vi "Simulated Database.vi"(11 "Command":T2) -> ()   [LabVIEW 2012]
uses:
  DataType/Simulated Database_Function.ctl
  DataType/Simulated Database_Record.ctl
panel:
  out "error out":errorcluster
  in  "error in (no error)":errorcluster
  out "owned record?":bool
  in  "Banlance or Account":i32
  out "Record":T1 {"Balance" format="%9.2f"; "Account Number" format="%0#5_5g"}
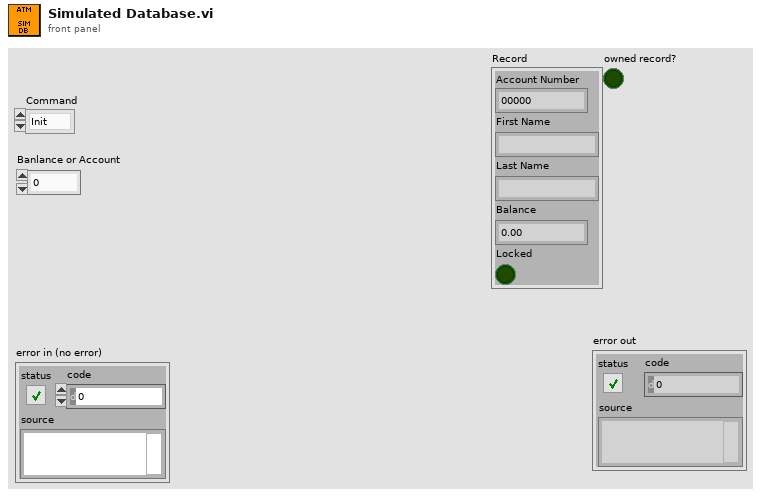
[diagram p1: front panel]
types:
  T1 = typedef "Simulated Database_Record.ctl" = cluster{"Account Number":dbl, "First Name":string, "Last Name":string, "Balance":dbl, "Locked":bool}
  T2 = typedef "Simulated Database_Function.ctl" = enum16{"Init", "Search account and lock record", "Modify balance", "Access record", "Commit record", "Unlock record", "Close"}
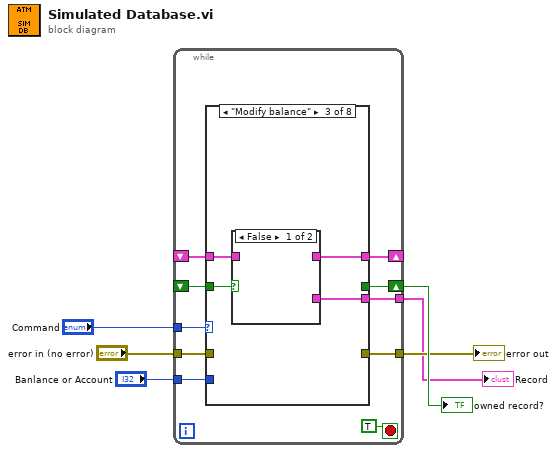
[diagram p0: block diagram]
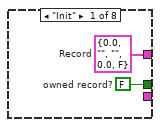
[diagram p2: hidden frame]
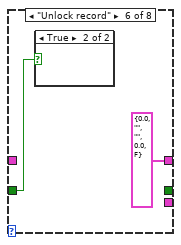
[diagram p10: hidden frame]
diagram:
  n1 = while {
    tunnel: "Command" -> [w15]
    shift-right: [w14] -> _
    shift-left: _ -> [w13]
    shift-right: [w12] -> w5
    shift-left: _ -> [w11]
    tunnel: [w10] -> w4
    tunnel: "error in (no error)" -> [w9]
    tunnel: "Banlance or Account" -> [w8]
    tunnel: [w7] -> w1
    stop <- TRUE stop-if-true
    n2 = case shown="\"Modify balance\"" w15 {
      tunnel: [w18 w21 w23 w28 w33 T1 {"Account Number"=0.0, "First Name"="", "Last Name"="", "Balance"=0.0, "Locked"=FALSE} ("Record") w39 w41] -> w14
      tunnel: w13 -> [_ w21 w24 w28 w33 _ w39 w41]
      tunnel: [w17 w20 _ _ w32 _ _ w40] -> w12
      tunnel: w11 -> [_ w20 w25 w30 w32 w37 _ w40]
      tunnel: [_ w19 _ w27 _ _ w38 w42] -> w10
      tunnel: w9 -> [_ w19 _ w27 _ _ w38 w42]
      tunnel: w8 -> [_ _ _ _ _ _ _ _]
      tunnel: [_ _ w22 w29 w34 _ _ _] -> w7
      frame "Init" {
        w17 = FALSE  # owned record?
        w18 = T1 {"Account Number"=0.0, "First Name"="", "Last Name"="", "Balance"=0.0, "Locked"=FALSE}  # Record
      }
      frame "Search account and lock record" {
        n3 = case shown="True" w20 {
          frame False {
          }
          frame True {
          }
        }
      }
      frame "Modify balance" {
        n4 = case shown="False" w25 {
          tunnel: [_ w26] -> w23
          tunnel: w24 -> [_ w26]
          tunnel: [_ w26] -> w22
          frame False {
          }
          frame True {
          }
        }
      }
      frame "Access record" {
        n5 = case shown="False" w30 {
          tunnel: [_ w31] -> w29
          tunnel: w28 -> [_ w31]
          frame False {
          }
          frame True {
          }
        }
      }
      frame "Commit record" {
        n6 = case shown="False" w32 {
          tunnel: [_ w35] -> w34
          tunnel: w33 -> [_ w35]
          frame False {
          }
          frame True {
          }
        }
      }
      frame "Unlock record" {
        n7 = case shown="True" w37 {
          frame False {
          }
          frame True {
          }
        }
      }
      frame "Close" {
      }
      frame Default {
      }
    }
  }
  "Record" <- w1
  "owned record?" <- w5
  "error out" <- w4
